vi "Connect.vi"(8 "error in (no error)":errorcluster, 11 "reference in":refnum<class "Camera_Sim.lvclass">) -> (0 "error out":errorcluster, 3 "reference out":refnum<class "Camera_Sim.lvclass">)   [LabVIEW 2017, in "Camera_Sim.lvclass"]
doc: "Connects to the IMAQ camera with the configured interface name. Returns error if connection unsuccessful."
uses:
  Camera_Sim.lvclass
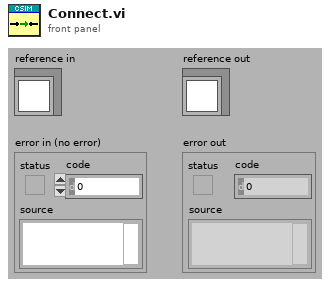
[diagram p1: front panel]
types:
  T1 = typedef "CameraSim.lvclass/ObjectAttributes.ctl" = cluster{"Connected":bool, "Image Out":T2, "Frame Number":u32, "Path":path}
  T2 = typedef "IMAQ Image.ctl" = refnum<image>
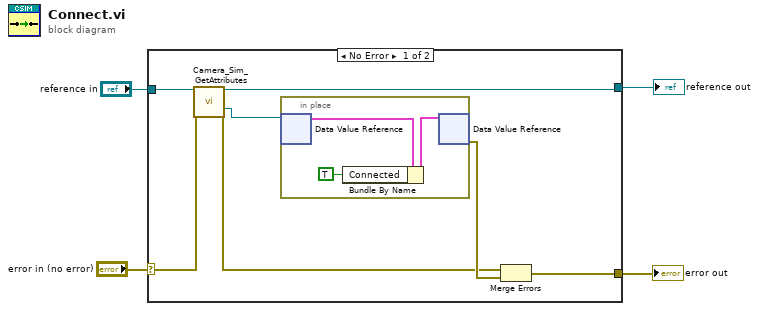
[diagram p0: block diagram]
diagram:
  n1 = case shown="No Error" "error in (no error)" {
    selector: "error in (no error)" -> [w10 w16]
    tunnel: [w7 w16] -> w3
    tunnel: [w5 w15] -> w1
    tunnel: "reference in" -> [w11 w15]
    frame No Error {
      n2 = call "Camera_Sim_GetAttributes.vi"("reference in"=w11, "error in (no error)"=w10) -> ("reference out"=w5:refnum<class "Camera_Sim.lvclass">, "DataRef"=w8:refnum<data-value>, "error out"=w6:errorcluster)  [unwired: 10 in, 1 out]
      n3 = in-place {
        n4 = in-place-dvr #1(w8) -> (w14:T1)  [unwired: 1 out]
        n5 = Bundle By Name(cluster=w14, "Connected"=TRUE) -> (w13:T1)
        n6 = in-place-dvr #1(w13) -> (w9:errorcluster)  [unwired: 1 out]
      }
      n7 = Merge Errors(w6, w9) -> (w7:errorcluster)
    }
    frame Error {
    }
  }
  "error out" <- w3
  "reference out" <- w1
